vi "Generate Header Vectors.vi"(0 "RFFE RegWriteExt Command in":refnum<class "RFFE RegWriteExt Command.lvclass">, 11 "error in (no error)":errorcluster) -> (4 "RFFE RegWriteExt Command out":refnum<class "RFFE RegWriteExt Command.lvclass">, 6 "Header Vectors":string[](array[string]), 15 "error out":errorcluster)   [LabVIEW 2018, in "MIPI RFFE API.lvlib" / "RFFE RegWriteExt Command.lvclass"]
uses:
  RFFE RegWriteExt Command.lvclass
  C:/Users/semoore/Projects/mipi-rffe-labview-oop/Extended Command/RFFE Extended Command.lvclass
  Extended Command/RFFE Extended Command.lvclass/RFFE Extended Command.ctl
  Extended Command/Get Register Data.vi
  Extended Command/RFFE Extended Command.lvclass
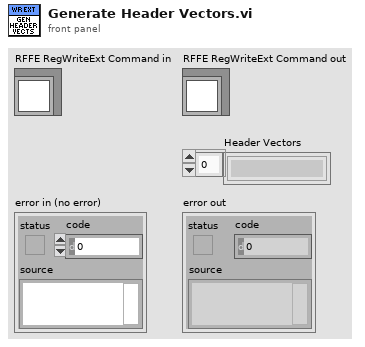
[diagram p1: front panel]
types:
  T1 = typedef "MIPI RFFE API.lvlib/Register Data.ctl" = u8
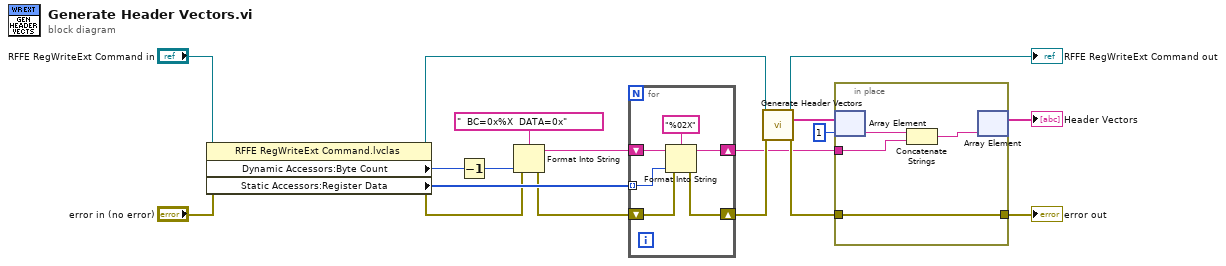
[diagram p0: block diagram]
diagram:
  n1 = property class="RFFE RegWriteExt Command.lvclas"(reference="RFFE RegWriteExt Command in", error in="error in (no error)") -> (reference out=w13:refnum<class "RFFE RegWriteExt Command.lvclass">, error out=w3:errorcluster, "Dynamic Accessors:Byte Count"=w6:i32, "Static Accessors:Register Data"=w4:T1[])
  n2 = Decrement(x=w6) -> (x-1=w1:i32)
  n3 = Format Into String(format string="  BC=0x%X  DATA=0x", error in=w3, w1) -> (resulting string=w7:string, error out=w2:errorcluster)  [unwired: 1 in]
  n4 = for {
    shift-right: [w19] -> w12
    shift-left: w2 -> [w20]
    tunnel: w4 -> [w24] mode=indexing
    shift-right: [w23] -> w10
    shift-left: w7 -> [w21]
    n5 = Format Into String(format string="%02X", initial string=w21, error in=w20, w24) -> (resulting string=w23:string, error out=w19:errorcluster)
  }
  n6 = call-parent "Generate Header Vectors.vi"("RFFE Command in"=w13, "error in (no error)"=w12) -> ("RFFE Command out"=→"RFFE RegWriteExt Command out":refnum<class "RFFE RegWriteExt Command.lvclass">, "Header Vectors"=w16:string[], "error out"=w15:errorcluster)  [unwired: 11 in]
  n7 = in-place {
    in-place-border: w15 -> [w25]
    in-place-border: w10 -> [w27]
    in-place-border: [w25] -> w8
    n8 = in-place-array #1(w16, 1) -> (w28:string)
    n9 = Concatenate Strings(w28, w27) -> (w26:string)
    n10 = in-place-array #1(w26) -> (→"Header Vectors":string[])  [unwired: 1 out]
  }
  "error out" <- w8
